vi "Initialize_Maj.vi"(8 "error in":errorcluster) -> (0 "error out":errorcluster)   [LabVIEW 2009]
uses:
  <vilib>/Utility/NIReport.llb/NI_report.lvclass
  <vilib>/Utility/NIReport.llb/HTML/NI_HTML.lvclass
  <instrlib>/Agilent 8000 Series/Agilent 8000 Series.lvlib
  <instrlib>/Agilent 81150/Agilent 81150.lvlib
panel:
  in  "Instrument VISA in":T1={"AWG VISA"="generadorpulsos", "Oscilloscope  VISA "="Oscilloscope", "Integration Board IP"="172.16.7.43", "connection ID"=refnum, "report out"=refnum, "report file path"=path "C:/Documents and Settings/CTA_LAB01/Desktop/L0_Asic/L0 Asic Test Data"}
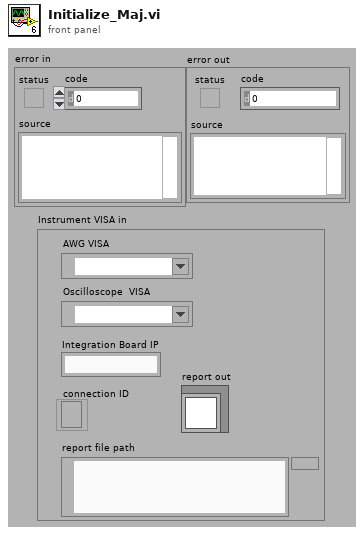
[diagram p1: front panel]
types:
  T1 = cluster{"AWG VISA":refnum<visa-resource-name>, "Oscilloscope  VISA ":refnum<visa-resource-name>, "Integration Board IP":string, "connection ID":refnum<k5>, "report out":refnum<class "NI_report.lvclass">, "report file path":path}
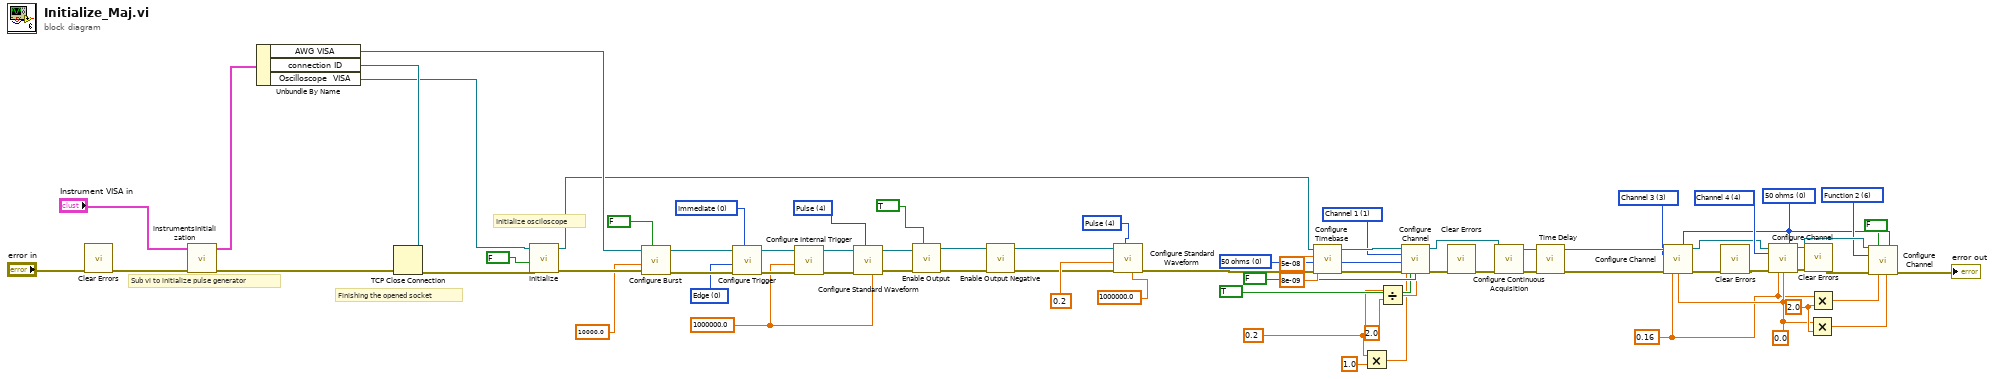
[diagram p0: block diagram]
diagram:
  w6 = u16 4 items=["Sine", "Square", "Ramp Up", "Ramp Down", "Pulse", "Noise", "DC"] ("Waveform (0: Sine)")
  w9 = 0.2 ("y")
  w11 = 0.16 ("Vertical Range (2.0 V)")
  w15 = 0.0 ("Vertical Offset (0.0 V)")
  w23 = 2.0 ("y")
  w17 = u32 0 items=["50 ohms", "1 Mohms"] ("Input Impedance (1: 1 Mohms)")
  w37 = u32 0 items=["50 ohms", "1 Mohms"] ("Input Impedance (1: 1 Mohms)")
  w40 = 1 items=["Channel 1"=1, "Channel 2"=2, "Channel 3"=3, "Channel 4"=4] ("Channel (1: Channel 1)")
  w27 = u16 6 items=["Function 1"=5, "Function 2"=6, "Function 3"=7, "Function 4"=8] ("Math Channel (5: Function 1)")
  w16 = 3 items=["Channel 1"=1, "Channel 2"=2, "Channel 3"=3, "Channel 4"=4] ("Channel (1: Channel 1)")
  w35 = 4 items=["Channel 1"=1, "Channel 2"=2, "Channel 3"=3, "Channel 4"=4] ("Channel (1: Channel 1)")
  w49 = 1000000.0 ("Frequency (1000.0 Hz)")
  w64 = u16 0 items=["Immediate", "Internal", "External", "Software Trigger Function"] ("Trigger Source (0: Immediate)")
  w65 = u16 0 items=["Edge", "Level"] ("Trigger Mode (0: Edge)")
  w68 = u16 4 items=["Sine", "Square", "Ramp Up", "Ramp Down", "Pulse", "Noise", "DC"] ("Waveform (0: Sine)")
  # "Initialize osciloscope"
  # "Finishing the opened socket"
  # "Sub vi to initialize pulse generator"
  n1 = call <vilib>:"Clear Errors.vi"("error in (no error)"="error in") -> ("error out"=w70:errorcluster)  [unwired: 6 in]
  n2 = call "instrumentsInitialization.vi"("error in"=w70, "Instrument VISA in"="Instrument VISA in") -> ("error out"=w58:errorcluster, "Instrument VISA out"=w2:T1)  [unwired: 8 in]
  n3 = Unbundle By Name(w2) -> ("AWG VISA"=w54:refnum<visa-resource-name>, "connection ID"=w59:refnum<k5>, "Oscilloscope  VISA"=w55:refnum<visa-resource-name>)
  n4 = TCP Close Connection(connection ID=w59, error in (no error)=w58) -> (error out=w53:errorcluster)  [unwired: 1 in, 1 out]
  n5 = call <instrlib>:"Initialize.vi"("error in (no error)"=w53, "Reset (True)"=FALSE ("ID Query (True)"), "VISA resource name"=w55) -> ("error out"=w46:errorcluster, "VISA resource name out"=w1:refnum<visa-resource-name>)  [unwired: 7 in]
  n6 = call <instrlib>:"Configure Burst.vi"("Enable Burst (F: Disable)"=FALSE, "error in (no error)"=w46, "Burst Count (2)"=10000.0 ("Frequency (1000.0 Hz)"), "VISA resource name"=w54) -> ("error out"=w67:errorcluster, "VISA resource name out"=w66:refnum<visa-resource-name>)  [unwired: 6 in]
  n7 = call <instrlib>:"Configure Trigger.vi"("Trigger Source (0: Immediate)"=w64, "error in (no error)"=w67, "Trigger Mode (0: Edge)"=w65, "VISA resource name"=w66) -> ("error out"=w63:errorcluster, "VISA resource name out"=w62:refnum<visa-resource-name>)  [unwired: 6 in]
  n8 = call <instrlib>:"Configure Internal Trigger.vi"("error in (no error)"=w63, "Frequency (100000.0 Hz)"=w49, "VISA resource name"=w62) -> ("error out"=w60:errorcluster, "VISA resource name out"=w61:refnum<visa-resource-name>)  [unwired: 7 in]
  n9 = call <instrlib>:"Configure Standard Waveform.vi"("Frequency (1000.0 Hz)"=w49, "Waveform (0: Sine)"=w68, "error in (no error)"=w60, "VISA resource name"=w61) -> ("error out"=w52:errorcluster, "VISA resource name out"=w51:refnum<visa-resource-name>)  [unwired: 6 in]
  n10 = call <instrlib>:"Enable Output.vi"("Enable Output (T: Enable)"=TRUE, "error in (no error)"=w52, "VISA resource name"=w51) -> ("error out"=w48:errorcluster, "VISA resource name out"=w47:refnum<visa-resource-name>)  [unwired: 7 in]
  n11 = call <instrlib>:"Enable Output Negative.vi"("error in (no error)"=w48, "VISA resource name"=w47) -> ("error out"=w4:errorcluster, "VISA resource name out"=w3:refnum<visa-resource-name>)  [unwired: 8 in]
  n12 = call <instrlib>:"Configure Standard Waveform.vi"("Frequency (1000.0 Hz)"=1000000.0, "Waveform (0: Sine)"=w6, "error in (no error)"=w4, "Amplitude (1.0 Vpp)"=0.2 ("y"), "VISA resource name"=w3) -> ("error out"=w5:errorcluster)  [unwired: 5 in, 1 out]
  n13 = call <instrlib>:"Configure Timebase.vi"("error in (no error)"=w5, "Position (0.0 s)"=8e-09, "Timebase (0.005 s)"=5e-08, "VISA resource name"=w1) -> ("error out"=w41:errorcluster, "VISA resource name out"=w42:refnum<visa-resource-name>)  [unwired: 6 in]
  n14 = Multiply(x=w9, y=1.0) -> (x*y=w24:dbl)
  n15 = Divide(x=w9, y=2.0) -> (x/y=w31:dbl)
  n16 = call <instrlib>:"Configure Channel.vi"("VISA resource name"=w42, "Enable Channel (Enable)"=TRUE, "BW Limit 20MHz (Disable)"=FALSE, "Input Impedance (1: 1 Mohms)"=w37, "Channel (1: Channel 1)"=w40, "error in (no error)"=w41, "Vertical Range (2.0 V)"=w24, "Vertical Offset (0.0 V)"=w31) -> ("VISA resource name out"=w14:refnum<visa-resource-name>, "error out"=w39:errorcluster)  [unwired: 6 in]
  n17 = call <vilib>:"Clear Errors.vi"("error in (no error)"=w39) -> ("error out"=w13:errorcluster)  [unwired: 6 in]
  n18 = call <instrlib>:"Configure Continuous Acquisition.vi"("error in (no error)"=w13, "VISA resource name"=w14) -> ("error out"=w26:errorcluster, "VISA resource name out"=w18:refnum<visa-resource-name>)  [unwired: 8 in]
  n19 = call "Time Delay"("error in (no error)"=w26) -> ("error out"=w19:errorcluster)  [unwired: 10 in]
  n20 = call <instrlib>:"Configure Channel.vi"("VISA resource name"=w18, "Input Impedance (1: 1 Mohms)"=w17, "Channel (1: Channel 1)"=w16, "error in (no error)"=w19, "Vertical Range (2.0 V)"=w11, "Vertical Offset (0.0 V)"=w15) -> ("VISA resource name out"=w20:refnum<visa-resource-name>, "error out"=w21:errorcluster)  [unwired: 8 in]
  n21 = call <vilib>:"Clear Errors.vi"("error in (no error)"=w21) -> ("error out"=w32:errorcluster)  [unwired: 6 in]
  n22 = call <instrlib>:"Configure Channel.vi"("VISA resource name"=w20, "Input Impedance (1: 1 Mohms)"=w17, "Channel (1: Channel 1)"=w35, "error in (no error)"=w32, "Vertical Range (2.0 V)"=w11, "Vertical Offset (0.0 V)"=w15) -> ("VISA resource name out"=w29:refnum<visa-resource-name>, "error out"=w33:errorcluster)  [unwired: 8 in]
  n23 = call <vilib>:"Clear Errors.vi"("error in (no error)"=w33) -> ("error out"=w30:errorcluster)  [unwired: 6 in]
  n24 = Multiply(x=w15, y=w23) -> (x*y=w22:dbl)
  n25 = Multiply(x=w11, y=w23) -> (x*y=w28:dbl)
  n26 = call <instrlib>:"Configure Channel.vi"("VISA resource name"=w29, "Enable Channel (Enable)"=FALSE, "Input Impedance (1: 1 Mohms)"=w17, "Channel (1: Channel 1)"=w27, "error in (no error)"=w30, "Vertical Range (2.0 V)"=w28, "Vertical Offset (0.0 V)"=w22) -> ("error out"=→"error out":errorcluster)  [unwired: 7 in, 1 out]
